vi "pinvTruncate.vi"(8 "error in (no error)":errorcluster, 9 "Truncation Threshold":dbl=0.0001, 10 "Matrix A":dbl[][](array[numeric]), 11 "MatOper in":refnum<class "MatOper.lvclass">) -> (0 "error out":errorcluster, 2 "Truncated Pinv A":dbl[][](array[numeric]), 3 "MatOper out":refnum<class "MatOper.lvclass">)   [LabVIEW 2016, in "MatOper.lvclass"]
doc: "Do the pseudo inverse with the truncation based on the threshold."
uses:
  MatOper.lvclass
  <vilib>/Analysis/baseanly.llb/Real A x B.vi
  <vilib>/Analysis/Matrix/Numeric/Conversions/Array To Matrix - RA2.vi
  <vilib>/Analysis/7linalg.llb/Real SVD Decomposition.vi
  <vilib>/Analysis/Matrix/Numeric/Conversions/Matrix To Array - RM.vi
  <vilib>/Analysis/NI_AALPro.lvlib
  <vilib>/Analysis/Matrix/NI_Matrix.lvlib
  <vilib>/Analysis/NI_AALBase.lvlib
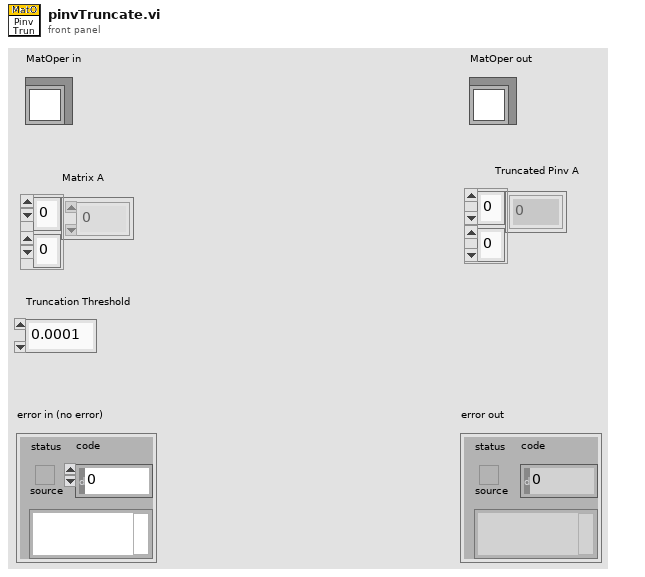
[diagram p1: front panel]
types:
  T1 = typedef "NI_Matrix.lvlib/RealMatrix.ctl" = dbl[][]
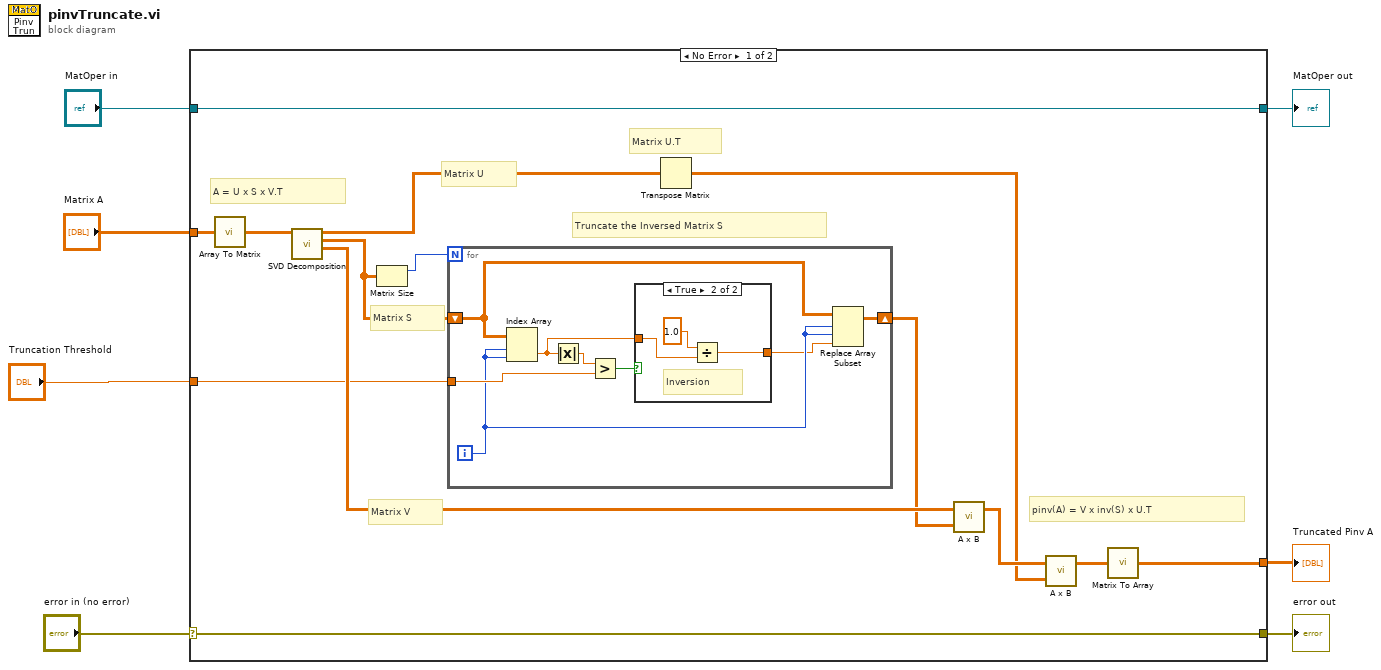
[diagram p0: block diagram]
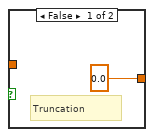
[diagram p2: hidden frame]
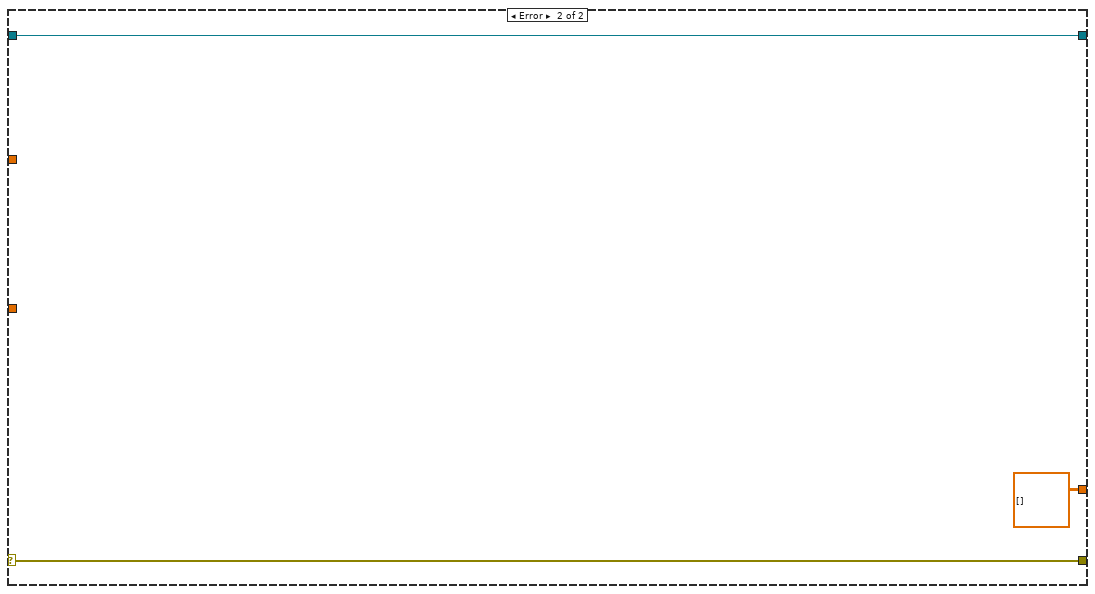
[diagram p3: hidden frame]
diagram:
  n1 = case shown="No Error" "error in (no error)" {
    selector: "error in (no error)" -> [w20 w36]
    tunnel: [w20 w36] -> w6
    tunnel: [w21 w35] -> w4
    tunnel: "MatOper in" -> [w21 w35]
    tunnel: "Truncation Threshold" -> [w10 _]
    tunnel: "Matrix A" -> [w9 _]
    tunnel: [w8 dbl[][] [] ("Real 2D Array")] -> w1
    frame No Error {
      # "pinv(A) = V x inv(S) x U.T"
      # "A = U x S x V.T"
      # "Matrix U"
      # "Matrix S"
      # "Truncate the Inversed Matrix S"
      # "Matrix U.T"
      # "Matrix V"
      n2 = call-poly <vilib>:"Array To Matrix.vi"("Real 2D Array"=w9) -> ("Real Matrix"=w19:T1)
      n3 = call-poly <vilib>:"SVD Decomposition.vi"("A"=w19) -> ("Matrix V"=w18:T1, "Matrix S"=w13:T1, "Matrix U"=w16:T1)  [unwired: 6 in, 2 out]
      n4 = Matrix Size(0:w13) -> (1:w14:i32)  [unwired: 1 out]
      n5 = for {
        N: w14 -> [_]
        tunnel: w10 -> [w28]
        shift-right: [w22] -> w12
        shift-left: w13 -> [w23]
        i -> [w25]
        n6 = Index Array(array=w23, index (row)=w25, index (col)=w25) -> (element=w26:dbl)
        n7 = Absolute Value(x=w26) -> (abs(x)=w29:dbl)
        n8 = Greater?(x=w29, y=w28) -> (0:w27:bool)
        n9 = case shown="True" w27 {
          tunnel: w26 -> [_ w32]
          tunnel: [0.0 w31] -> w24
          frame False {
            # "Truncation"
          }
          frame True {
            # "Inversion"
            n10 = Divide(x=1.0, y=w32) -> (x/y=w31:dbl)
          }
        }
        n11 = Replace Array Subset(array=w23, new element=w24, index (row)=w25, index (col)=w25) -> (w22:T1)
      }
      n12 = Transpose Matrix(1:w16) -> (0:w15:T1)
      n13 = call-poly <vilib>:"A x B.vi"("B"=w12, "A"=w18) -> ("A x B"=w17:T1)  [unwired: 1 out]
      n14 = call-poly <vilib>:"A x B.vi"("B"=w15, "A"=w17) -> ("A x B"=w11:T1)  [unwired: 1 out]
      n15 = call-poly <vilib>:"Matrix To Array.vi"("Real Matrix"=w11) -> ("Real 2D Array"=w8:dbl[][])
    }
    frame Error {
    }
  }
  "error out" <- w6
  "MatOper out" <- w4
  "Truncated Pinv A" <- w1
